vi "Rvp8XmlCommands.vi"(1 "nGates":u16=500 min=1025 step=1, 2 "startGate":u16=50 min=1025 step=1, 3 "nSamples":i32=1000) -> (0 "TsGrabberCommand":string)   [LabVIEW 2009]
doc: "Sends an XML command to an instrument.\nWaits for the reply.\nReply string must end in specified string."
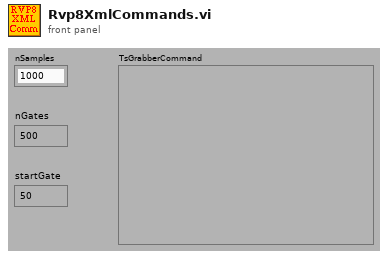
[diagram p1: front panel]
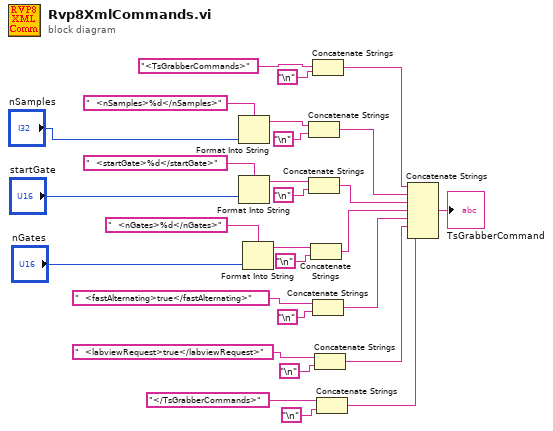
[diagram p0: block diagram]
diagram:
  n1 = Format Into String(format string="  <nSamples>%d</nSamples>", "nSamples") -> (resulting string=w12:string)  [unwired: 2 in, 1 out]
  n2 = Format Into String(format string="  <startGate>%d</startGate>", "startGate") -> (resulting string=w11:string)  [unwired: 2 in, 1 out]
  n3 = Format Into String(format string="  <nGates>%d</nGates>", "nGates") -> (resulting string=w10:string)  [unwired: 2 in, 1 out]
  n4 = Concatenate Strings(w12, "\n") -> (w6:string)
  n5 = Concatenate Strings(w11, "\n") -> (w5:string)
  n6 = Concatenate Strings(w10, "\n") -> (w4:string)
  n7 = Concatenate Strings("<TsGrabberCommands>" ("format string"), "\n") -> (w19:string)
  n8 = Concatenate Strings("  <fastAlternating>true</fastAlternating>", "\n") -> (w3:string)
  n9 = Concatenate Strings("  <labviewRequest>true</labviewRequest>" ("format string"), "\n") -> (w2:string)
  n10 = Concatenate Strings("</TsGrabberCommands>" ("format string"), "\n") -> (w1:string)
  n11 = Concatenate Strings(w19, w6, w5, w4, w3, w2, w1) -> (→"TsGrabberCommand":string)
